vi "ConfigureWaveforms.vi"(0 "WFReferences":T1, 1 "PreLoad Charts?":bool=TRUE, 5 "path":path=path "C:/Users/lab-341/Desktop/Reed/Oscilloscope VI/SlowCtrlRecent.bin", 11 "Iteration Duration":i64) -> ()   [LabVIEW 2012]
uses:
  TypeDefs/DataTypes/SlowCtrlRecent.ctl
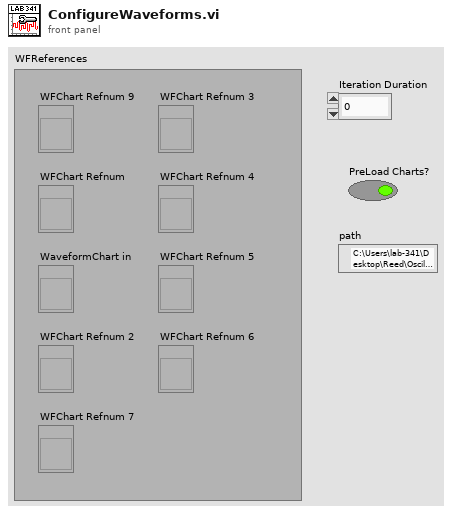
[diagram p1: front panel]
types:
  T1 = cluster{"WFChart Refnum":refnum<vi>, "WFChart Refnum 2":refnum<vi>, "WFChart Refnum 3":refnum<vi>, "WFChart Refnum 4":refnum<vi>, "WFChart Refnum 5":refnum<vi>, "WFChart Refnum 6":refnum<vi>, "WFChart Refnum 7":refnum<vi>, "WaveformChart in":refnum<vi>, "WFChart Refnum 9":refnum<vi>}
  T2 = typedef "SlowCtrlRecent.ctl" = cluster{"seconds since 1Jan1904":timestamp, "History Data":dbl[][], "LXe":dbl}
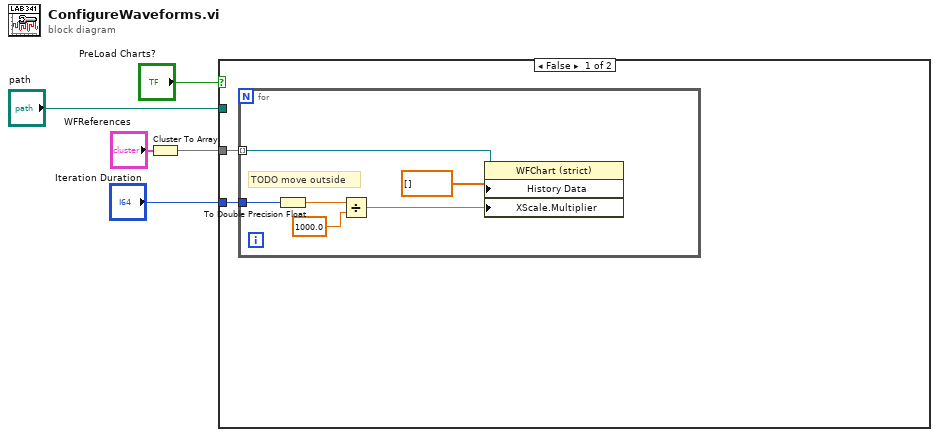
[diagram p0: block diagram]
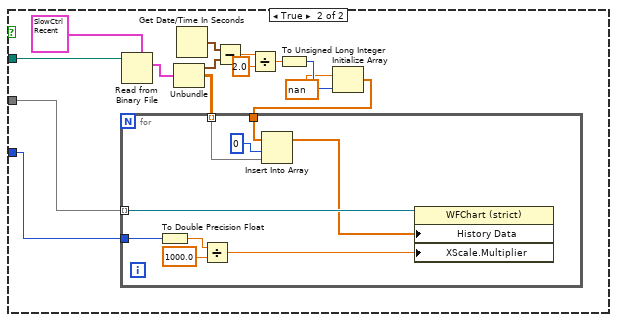
[diagram p2: hidden frame]
diagram:
  n1 = Cluster To Array(cluster="WFReferences") -> (array=w4:refnum<vi>[])
  n2 = case shown="False" "PreLoad Charts?" {
    tunnel: w4 -> [w7 w27]
    tunnel: "Iteration Duration" -> [w6 w26]
    tunnel: "path" -> [_ w25]
    frame False {
      n3 = for {
        tunnel: w7 -> [w12] mode=indexing
        tunnel: w6 -> [w11]
        # "TODO move outside"
        n4 = To Double Precision Float(number=w11) -> (double precision float=w9:dbl)
        n5 = Divide(x=w9, y=1000.0) -> (x/y=w10:dbl)
        n6 = property on="Property Node" class="WFChart (strict)"(reference=w12, "History Data"=dbl[] [], "XScale.Multiplier"=w10) -> ()  [unwired: 1 in, 2 out]
      }
    }
    frame True {
      n7 = Read from Binary File(5:T2 {"seconds since 1Jan1904"=timestamp(0 s since 1904-01-01), "History Data"=[], "LXe"=0.0} ("output cluster"), 11:w25) -> (2:w24:T2)  [unwired: 4 in, 3 out]
      n8 = Unbundle(w24) -> ("seconds since 1Jan1904"=w22:timestamp, "History Data"=w21:dbl[][])  [unwired: 1 out]
      n9 = Get Date/Time In Seconds() -> (seconds since 1Jan1904=w23:timestamp)
      n10 = Subtract(x=w23, y=w22) -> (x-y=w19:dbl)
      n11 = Divide(x=w19, y=2.0) -> (x/y=w18:dbl)
      n12 = To Unsigned Long Integer(number=w18) -> (unsigned 32bit integer=w17:u32)
      n13 = Initialize Array(nan, w17) -> (w15:dbl[])
      n14 = for {
        tunnel: w26 -> [w36]
        tunnel: w27 -> [w32] mode=indexing
        tunnel: w21 -> [w29] mode=indexing
        tunnel: w15 -> [w28]
        n15 = To Double Precision Float(number=w36) -> (double precision float=w34:dbl)
        n16 = Divide(x=w34, y=1000.0) -> (x/y=w35:dbl)
        n17 = Insert Into Array(array=w28, index=0, new element=w29) -> (w30:dbl[])
        n18 = property on="Property Node" class="WFChart (strict)"(reference=w32, "History Data"=w30, "XScale.Multiplier"=w35) -> ()  [unwired: 1 in, 2 out]
      }
    }
  }
